vi "Do Mutate.vi"(8 "error in":errorcluster, 10 "IGene in":refnum<class "IGene.lvclass">, 11 "Real Mutator in":refnum<class "Real Mutator.lvclass">) -> (0 "error out":errorcluster, 2 "IGene out":refnum<class "IGene.lvclass">, 3 "Real Mutator out":refnum<class "Real Mutator.lvclass">)   [LabVIEW 2016, in "Real Mutator.lvclass"]
doc: "This VI performs mutation of a Real Gene by <B>adding (+) a Mutation Delta</B> (specified by Real Mutator:Mutation Delta parameter). \nThe Mutation Delta is a random value normally distributed on a [Upper,Lower] interval.\nThis VI is a DD-override of the <B>Mutator:Do Mutate</B> method for Real-valued genes.\n\n**Author: Stas Legedza"
uses:
  Real Mutator.lvclass
  C:/Users/J51654/My Projects/Evolutionary Programming/GA Framework/GA Core/GA Core.lvclass
  IGene/IGene.lvclass
  GA Core.lvclass/GA Core.ctl
  IGene/Children/RealVal/Real Gene.lvclass
  C:/Users/J51654/My Projects/Evolutionary Programming/GA Framework/IGene/IGene.lvclass
  Real Mutator.lvclass/Real Mutator.ctl
  IGene/Children/RealVal/Real Gene.lvclass/Real Gene.ctl
  <vilib>/Utility/error.llb/Error Cluster From Error Code.vi
  <vilib>/ErrorRing/Error Ring.xnode
  GA Core.lvclass
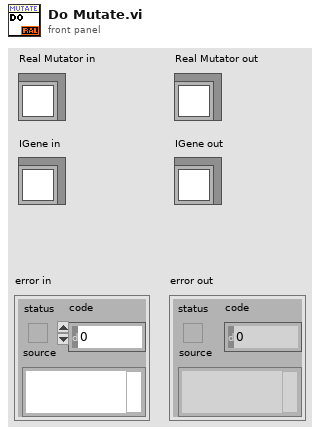
[diagram p1: front panel]
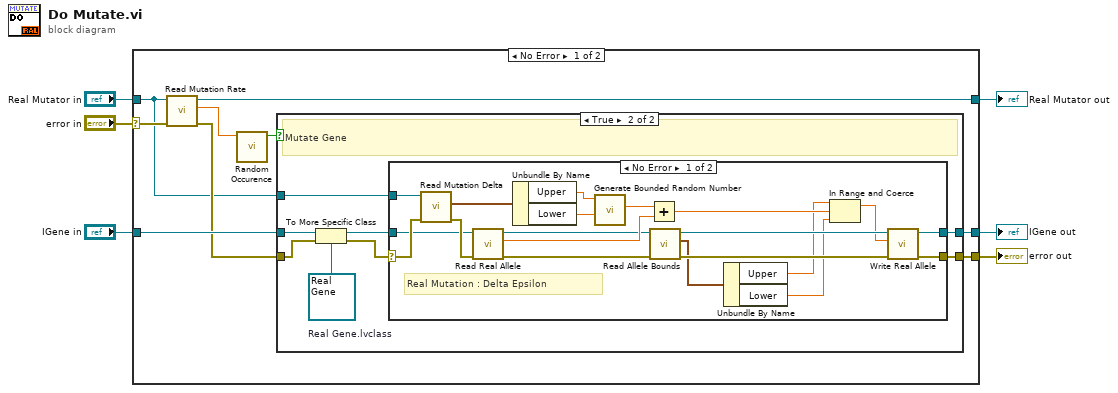
[diagram p0: block diagram]
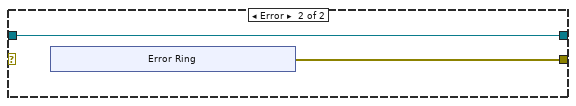
[diagram p3: hidden frame]
diagram:
  n1 = case shown="No Error" "error in" {
    selector: "error in" -> [w13 w54]
    tunnel: "Real Mutator in" -> [w7 w55]
    tunnel: "IGene in" -> [w14 w53]
    tunnel: [w15 w55] -> w3
    tunnel: [w11 w54] -> w1
    tunnel: [w10 w53] -> w2
    frame No Error {
      n2 = call "Read Mutation Rate.vi"("error in (no error)"=w13, "GA Core in"=w7) -> ("error out"=w12:errorcluster, "Mutation Rate"=w9:dbl, "GA Core out"=w15:refnum<class "Real Mutator.lvclass">)  [unwired: 7 in]
      n3 = call "Random Occurence.vi"("Probability of Occurence (0-1)"=w9) -> ("Occured?"=w8:bool)  [unwired: 10 in]
      n4 = case shown="True" w8 {
        tunnel: w14 -> [w17 w25]
        tunnel: w12 -> [w16 w22]
        tunnel: [w16 w21] -> w11
        tunnel: [w17 w20] -> w10
        tunnel: w7 -> [_ w18]
        frame False {
          # "Mutation did not occur"
        }
        frame True {
          w19 = refnum<class "Real Gene.lvclass"> refnum  # Real Gene.lvclass
          # "Mutate Gene"
          n5 = To More Specific Class(target class=w19, reference=w25, error in=w22) -> (specific class reference=w24:refnum<class "Real Gene.lvclass">, error out=w23:errorcluster)
          n6 = case shown="No Error" w23 {
            selector: w23 -> [w43 _]
            tunnel: w24 -> [w41 w46]
            tunnel: [w44 w47] -> w21
            tunnel: [w45 w46] -> w20
            tunnel: w18 -> [w40 _]
            frame No Error {
              # "Real Mutation : Delta Epsilon"
              n7 = call "Read Mutation Delta.vi"("error in (no error)"=w43, "Real Mutator in"=w40) -> ("error out"=w42:errorcluster, "Mutation Delta"=w39:cluster{"Upper":dbl, "Lower":dbl})  [unwired: 7 in, 1 out]
              n8 = call "Read Real Allele.vi"("error in (no error)"=w42, "Real Gene in"=w41) -> ("error out"=w32:errorcluster, "Real Allele"=w35:dbl, "Real Gene out"=w33:refnum<class "Real Gene.lvclass">)  [unwired: 7 in]
              n9 = Unbundle By Name(w39) -> ("Upper"=w38:dbl, "Lower"=w37:dbl)
              n10 = call "Generate Bounded Random Number.vi"("Lower (0.00)"=w37, "Upper (1.00)"=w38) -> ("Random Number"=w36:dbl)  [unwired: 9 in]
              n11 = Add(x=w36, y=w35) -> (x+y=w34:dbl)
              n12 = call "Read Allele Bounds.vi"("error in (no error)"=w32, "Real Gene in"=w33) -> ("error out"=w31:errorcluster, "Allele Bounds"=w29:cluster{"Upper":dbl, "Lower":dbl}, "Real Gene out"=w30:refnum<class "Real Gene.lvclass">)  [unwired: 7 in]
              n13 = Unbundle By Name(w29) -> ("Upper"=w28:dbl, "Lower"=w27:dbl)
              n14 = In Range and Coerce(upper limit=w28, x=w34, lower limit=w27) -> (coerced(x)=w26:dbl)  [unwired: 1 out]
              n15 = call "Write Real Allele.vi"("error in (no error)"=w31, "Real Allele"=w26, "Real Gene in"=w30) -> ("error out"=w44:errorcluster, "Real Gene out"=w45:refnum<class "Real Gene.lvclass">)  [unwired: 7 in]
            }
            frame Error {
              n16 = xnode "Error Ring"() -> ("error out"=w47:errorcluster)
            }
          }
        }
      }
    }
    frame Error {
    }
  }
  "error out" <- w1
  "Real Mutator out" <- w3
  "IGene out" <- w2
